vi "log in alpha.vi"() -> ()   [LabVIEW 2013]
panel:
  out "String":string="right"
  out "pass/fail":bool
  in  "stop":bool
  in  "OK Button":bool
  in  "Password":string
  in  "User name":string
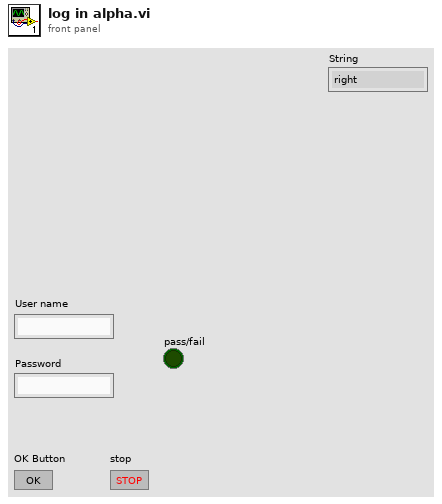
[diagram p1: front panel]
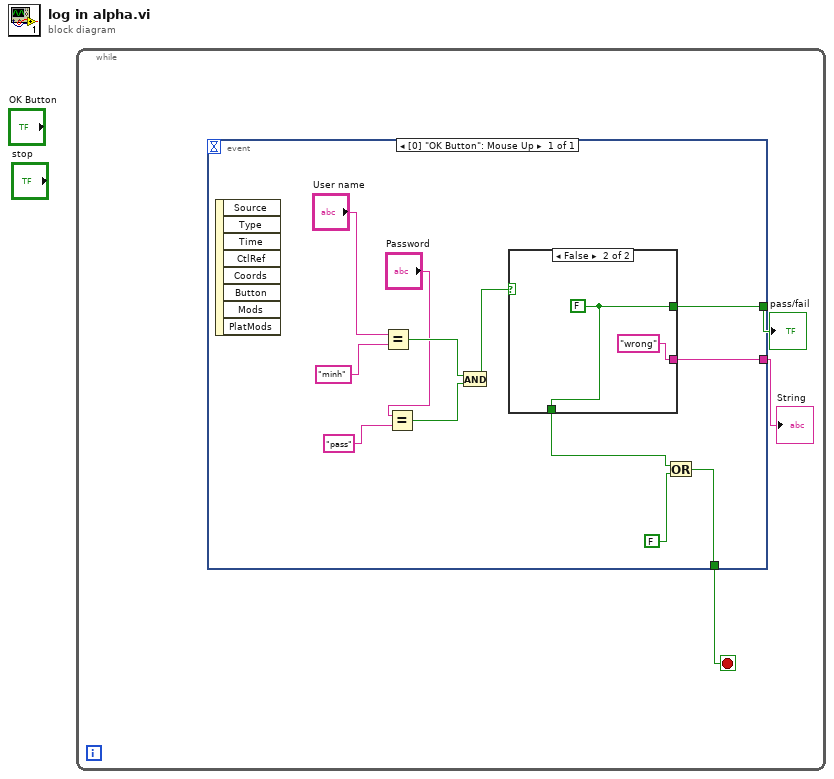
[diagram p0: block diagram]
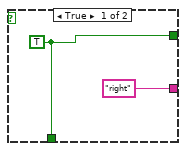
[diagram p2: hidden frame]
diagram:
  n1 = while {
    stop <- w3 stop-if-true
    n2 = event shown="[0] \"OK Button\": Mouse Up" {
      selector: _ -> [_]
      dyn-events: _ -> [_]
      timeout: _ -> [_]
      tunnel: [w8] -> w3
      tunnel: [w7] -> w2
      tunnel: [w6] -> w1
      event "OK Button": Mouse Up {
        n3 = event-data() -> ()  [unwired: 1 in, 8 out]
        n4 = Equal?(x="User name", y="minh" ("User name")) -> (x = y?=w13:bool)
        n5 = Equal?(x="Password", y="pass" ("Password")) -> (x = y?=w12:bool)
        n6 = And(x=w13, y=w12) -> (x .and. y?=w11:bool)
        n7 = case shown="False" w11 {
          tunnel: [w17 w19] -> w10
          tunnel: [w17 w19] -> w7
          tunnel: ["right" "wrong"] -> w6
          frame True {
            w17 = TRUE ("x .and. y?")
          }
          frame False {
            w19 = FALSE ("x .and. y?")
          }
        }
        n8 = Or(x=w10, y=FALSE) -> (x .or. y?=w8:bool)
      }
    }
    "pass/fail" <- w2
    "String" <- w1
  }
